vi "TabControl.vi"() -> ()   [LabVIEW 2016, in "test_ValueSignal.lvlib"]
uses:
  test_ValueSignal.lvlib
  Helper/HelperVI1.vi
  main/apis/Setup/GetVI/GetVIByPath.vi
  main/apis/Stimulus/ValueSignal/ValueSignalByPathString.vi
  main/apis/Assert/AssertControlValue/True.vi
  main/apis/Assert/AssertControlValue/Equal.vi
  main/Drona.lvlib
  main/apis/Stimulus/ValueSignal/ValueSignal.lvlib
  main/apis/Setup/GetVI/GetVI.lvlib
  <vilib>/addons/_JKI Toolkits/Caraya/classes/Test/Test.lvclass
  main/apis/Assert/AssertControlValue/AssertControlValue.lvlib
panel:
  out "error out":errorcluster
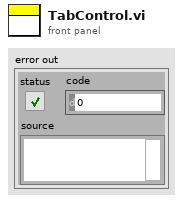
[diagram p1: front panel]
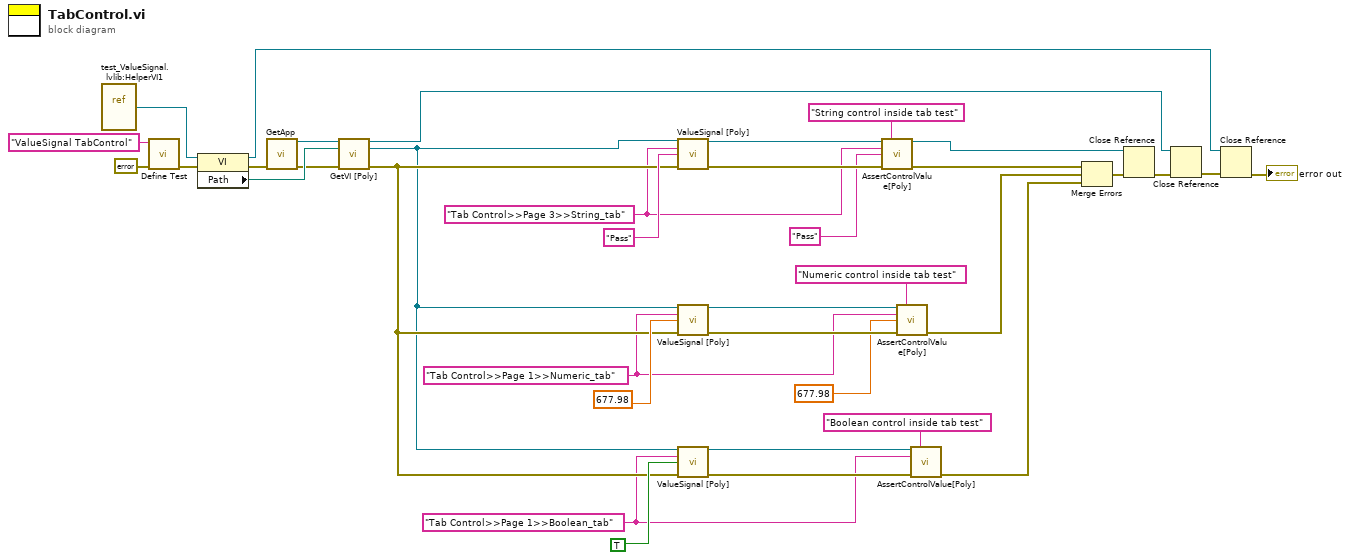
[diagram p0: block diagram]
diagram:
  w1 = "Tab Control>>Page 1>>Boolean_tab" ("Control Name")
  w2 = "Tab Control>>Page 1>>Numeric_tab" ("Control Name")
  w3 = "Tab Control>>Page 3>>String_tab" ("Control Name")
  n1 = vi-ref "test_ValueSignal.lvlib:HelperVI1.vi"() -> (w4:refnum<vi>)
  n2 = call <vilib>:"Define Test.vi"("error in (no error)"=errorcluster {"status"=FALSE, "code"=0, "source"=""}, "Label (VI Title)"="ValueSignal TabControl") -> ("error out"=w26:errorcluster)  [unwired: 9 in]
  n3 = property on="Property Node" class="VI"(reference=w4, error in=w26) -> (reference out=w21:refnum<vi>, error out=w30:errorcluster, "Path"=w29:path)
  n4 = call "GetApp.vi"("error in (no error)"=w30) -> ("Application Ref"=w31:refnum<vi>, "error out"=w28:errorcluster)  [unwired: 13 in]
  n5 = call-poly "GetVI [Poly].vi"("Application Ref in"=w31, "VI Path"=w29, "error in (no error)"=w28) -> ("Application Ref out"=w22:refnum<vi>, "VI Reference"=w23:refnum<vi>, "error out"=w24:errorcluster)  [unwired: 10 in]
  n6 = call-poly "ValueSignal [Poly].vi"("VI Reference In"=w23, "Control Name"=w3, "Value (Signaling)"="Pass" ("Control Name"), "error in"=w24) -> ("VI Reference Out"=w18:refnum<vi>, "error out"=w20:errorcluster)  [unwired: 10 in]
  n7 = call-poly "ValueSignal [Poly].vi"("VI Reference In"=w23, "Control Name"=w2, "Value (Signaling)"=677.98, "error in"=w24) -> ("VI Reference Out"=w12:refnum<vi>, "error out"=w14:errorcluster)  [unwired: 10 in]
  n8 = call-poly "ValueSignal [Poly].vi"("VI Reference In"=w23, "Control Name"=w1, "Value (Signaling)"=TRUE, "error in"=w24) -> ("VI Reference Out"=w7:refnum<vi>, "error out"=w9:errorcluster)  [unwired: 10 in]
  n9 = call-poly "AssertControlValue[Poly].vi"("VI Reference In"=w18, "Label"="String control inside tab test" ("Label (VI Title)"), "Control Name"=w3, "Control Value"="Pass" ("Control Name"), "Error In"=w20) -> ("VI Reference Out"=w16:refnum<vi>, "Error Out"=w19:errorcluster)  [unwired: 9 in]
  n10 = call-poly "AssertControlValue[Poly].vi"("VI Reference In"=w12, "Label"="Numeric control inside tab test" ("Label (VI Title)"), "Control Name"=w2, "Control Value"=677.98, "Error In"=w14) -> ("Error Out"=w13:errorcluster)  [unwired: 9 in, 1 out]
  n11 = call-poly "AssertControlValue[Poly].vi"("VI Reference In"=w7, "Label"="Boolean control inside tab test" ("Label (VI Title)"), "Control Name"=w1, "Error In"=w9) -> ("Error Out"=w8:errorcluster)  [unwired: 10 in, 1 out]
  n12 = Merge Errors(w19, w13, w8) -> (w34:errorcluster)
  n13 = Close Reference(reference=w16, error in (no error)=w34) -> (error out=w36:errorcluster)
  n14 = Close Reference(reference=w22, error in (no error)=w36) -> (error out=w35:errorcluster)
  n15 = Close Reference(reference=w21, error in (no error)=w35) -> (error out=→"error out":errorcluster)
